vi "Pack Data.vi"(5 "Math":T3, 6 "Encoder":T2) -> (0 "RR Data":T1, 1 "RL Data":T1, 2 "FL Data":T1, 3 "FR Data":T1)   [LabVIEW 2018]
uses:
  Motor Data Unpacked.ctl
  Encoder Unpacked Data.ctl
  Final Motor Data.ctl
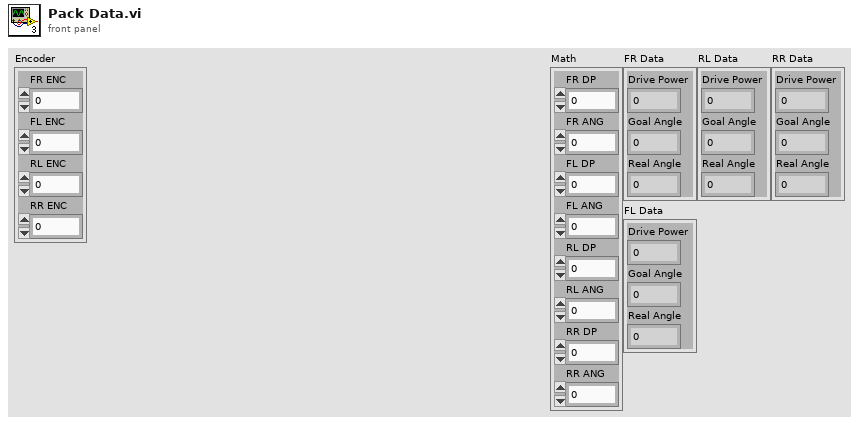
[diagram p1: front panel]
types:
  T1 = typedef "Final Motor Data.ctl" = cluster{"Drive Power":dbl, "Goal Angle":dbl, "Real Angle":dbl}
  T2 = typedef "Encoder Unpacked Data.ctl" = cluster{"FR ENC":dbl, "FL ENC":dbl, "RL ENC":dbl, "RR ENC":dbl}
  T3 = typedef "Motor Data Unpacked.ctl" = cluster{"FR DP":dbl, "FR ANG":dbl, "FL DP":dbl, "FL ANG":dbl, "RL DP":dbl, "RL ANG":dbl, "RR DP":dbl, "RR ANG":dbl}
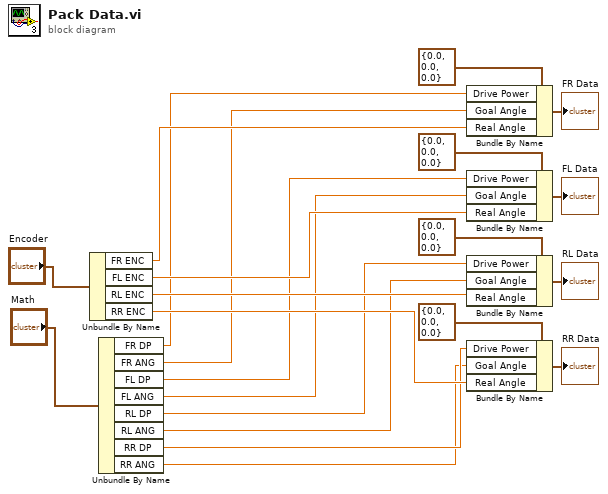
[diagram p0: block diagram]
diagram:
  n1 = Unbundle By Name("Encoder") -> ("FR ENC"=w16:dbl, "FL ENC"=w15:dbl, "RL ENC"=w14:dbl, "RR ENC"=w13:dbl)
  n2 = Unbundle By Name("Math") -> ("FR DP"=w12:dbl, "FR ANG"=w10:dbl, "FL DP"=w11:dbl, "FL ANG"=w9:dbl, "RL DP"=w8:dbl, "RL ANG"=w7:dbl, "RR DP"=w6:dbl, "RR ANG"=w5:dbl)
  n3 = Bundle By Name(cluster=T1 {"Drive Power"=0.0, "Goal Angle"=0.0, "Real Angle"=0.0}, "Drive Power"=w12, "Goal Angle"=w10, "Real Angle"=w16) -> (→"FR Data":T1)
  n4 = Bundle By Name(cluster=T1 {"Drive Power"=0.0, "Goal Angle"=0.0, "Real Angle"=0.0}, "Drive Power"=w11, "Goal Angle"=w9, "Real Angle"=w15) -> (→"FL Data":T1)
  n5 = Bundle By Name(cluster=T1 {"Drive Power"=0.0, "Goal Angle"=0.0, "Real Angle"=0.0}, "Drive Power"=w8, "Goal Angle"=w7, "Real Angle"=w14) -> (→"RL Data":T1)
  n6 = Bundle By Name(cluster=T1 {"Drive Power"=0.0, "Goal Angle"=0.0, "Real Angle"=0.0}, "Drive Power"=w6, "Goal Angle"=w5, "Real Angle"=w13) -> (→"RR Data":T1)
